vi "STM Set Meta Data (TCP Clst).vi"(7 "Meta data":T2[](array[typedef]), 8 "error in":errorcluster, 11 "Connection Info In":T1) -> (0 "error out":errorcluster, 3 "Connection Info Out":T1)   [LabVIEW 2013]
doc: "Assigns the meta data cluster associated with this STM session."
uses:
  stm_TCP Connection Info.ctl
  stm_MetaDataElement.ctl
  NI STM.lvlib
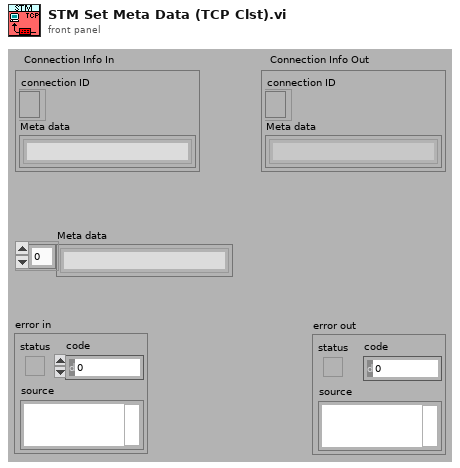
[diagram p1: front panel]
types:
  T1 = typedef "stm_TCP Connection Info.ctl" = cluster{"connection ID":refnum<k5>, "Meta data":T2[]}
  T2 = typedef "stm_MetaDataElement.ctl" = string
  T3 = typedef "NI STM.lvlib/TCP Connection Info.ctl" = cluster{"connection ID":refnum<k5>, "meta data":T4[]}
  T4 = typedef "NI STM.lvlib/MetaDataElement.ctl" = string
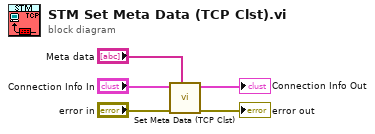
[diagram p0: block diagram]
diagram:
  n1 = call "Set Meta Data (TCP Clst).vi"("meta data"="Meta data", "error in"="error in", "connection info in"="Connection Info In") -> ("error out"=→"error out":errorcluster, "connection info out"=→"Connection Info Out":T3)  [unwired: 7 in]
